vi "Constants.vi"() -> ()   [LabVIEW 2014, in "OPC UA Client Shared.lvlib"]
doc: "Use this Global VI to access the GUIDs assigned to the page resources of the Custom Device."
uses:
  OPC UA Client Shared.lvlib
panel:
  in  "Tab Control":enum32{"GUIDS", "Constants", "Properties"}(tab)
  in  "Update Rate":string="ed5bc354-1ea5-4a40-a6d4-2ade4b72cc1c"
  in  "Status":string="7edfa8db-1108-4455-b477-d5a5949050b3"
  in  "Node":string="516c300a-dfa6-4a3e-922a-bc0c1d57111b"
  in  "Access":string="fa925dd1-b257-49c9-ad11-0163bcbdb07b"
  in  "OPC UA Client":string="b427fdee-6f3d-4280-85b2-59e4741516b9"
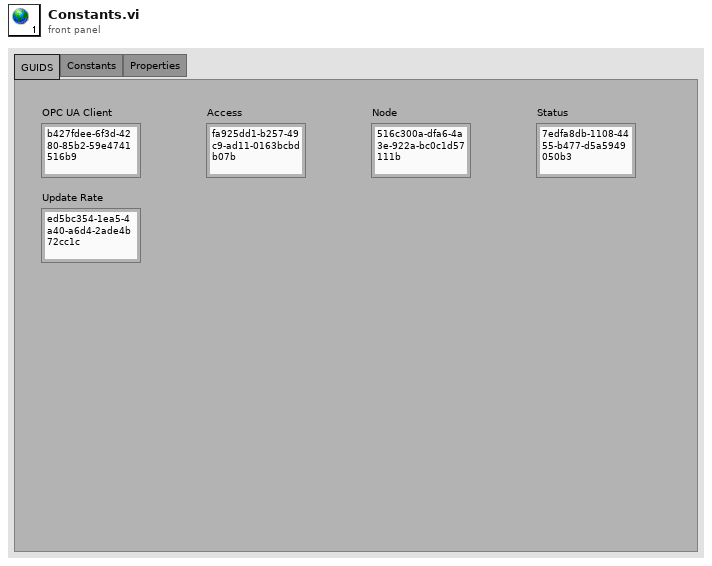
[diagram p1: front panel]
diagram:
